vi "Enqueue Element String.vi"(6 "High Priority?(F)":bool, 8 "error in (no error)":errorcluster, 9 "timeout in ms (-1)":i32, 10 "CSM Timestamp Argument":string, 11 "Priority Queue":refnum<class "Priority Queue.lvclass">) -> (0 "error out":errorcluster, 3 "Priority Queue":refnum<class "Priority Queue.lvclass">)   [LabVIEW 2014, in "Communicable State Machine.lvlib" / "Priority Queue.lvclass"]
uses:
  Priority Queue.lvclass
  Priority Queue.lvclass/Priority Queue.ctl
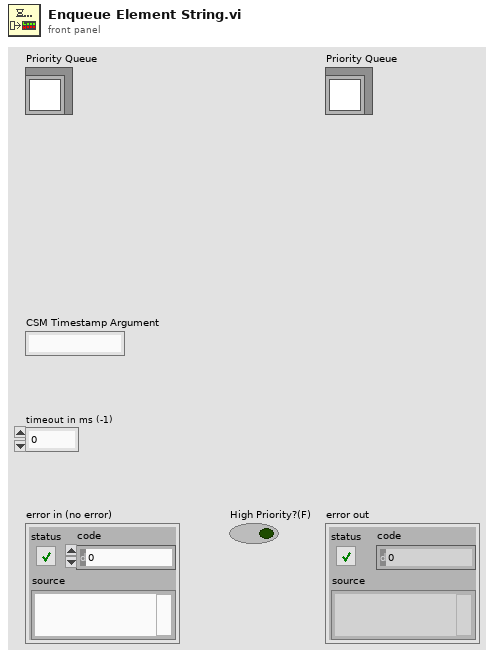
[diagram p1: front panel]
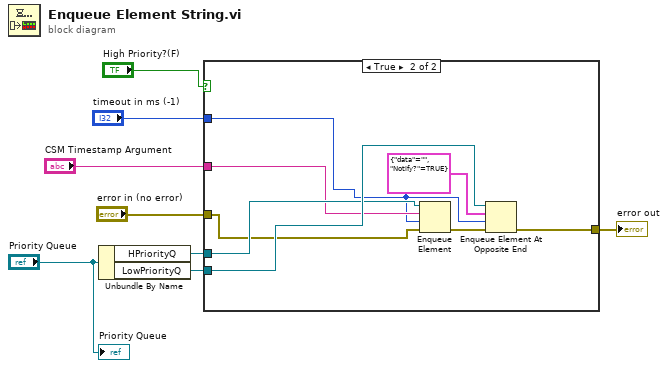
[diagram p0: block diagram]
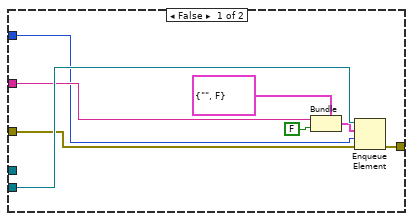
[diagram p2: hidden frame]
diagram:
  n1 = Unbundle By Name("Priority Queue") -> ("HPriorityQ"=w6:refnum<queue>, "LowPriorityQ"=w5:refnum<queue>)
  n2 = case shown="True" "High Priority?(F)" {
    tunnel: w5 -> [w16 w24]
    tunnel: "CSM Timestamp Argument" -> [w15 w22]
    tunnel: w6 -> [_ w23]
    tunnel: "error in (no error)" -> [w11 w19]
    tunnel: [w10 w21] -> w8
    tunnel: "timeout in ms (-1)" -> [w9 w20]
    frame False {
      n3 = Bundle(cluster=cluster{"data":string, "Notify?":bool} {"data"="", "Notify?"=FALSE}, "data"=w15, "Notify?"=FALSE) -> (w12:cluster{"data":string, "Notify?":bool})
      n4 = Enqueue Element(queue=w16, element=w12, timeout in ms (-1)=w9, error in (no error)=w11) -> (error out=w10:errorcluster)  [unwired: 2 out]
    }
    frame True {
      n5 = Enqueue Element(queue=w23, element=w22, timeout in ms (-1)=w20, error in (no error)=w19) -> (error out=w18:errorcluster)  [unwired: 2 out]
      n6 = Enqueue Element At Opposite End(queue=w24, element=cluster{"data":string, "Notify?":bool} {"data"="", "Notify?"=TRUE} ("cluster"), timeout in ms (-1)=w20, error in (no error)=w18) -> (error out=w21:errorcluster)  [unwired: 2 out]
    }
  }
  "error out" <- w8
  "Priority Queue" <- "Priority Queue"
